vi "Mystery VI.vi"(4 "Old X-Axis":i32, 6 "Old Pin":bool[](array[boolean]), 7 "X-Axis":i32, 9 "Pin":bool[](array[boolean]), 10 "Old Trace":bool[](array[boolean]), 11 "Trace":bool[](array[boolean])) -> (1 "Updated X-Axis":i32, 2 "Updated Old Pin?":bool[](array[boolean]), 3 "NeedUpdate?":bool, 5 "Updated Old Trace?":bool[](array[boolean]))   [LabVIEW 2019]
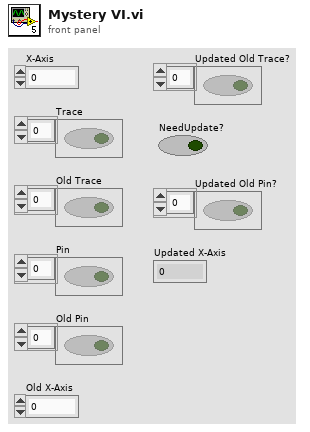
[diagram p1: front panel]
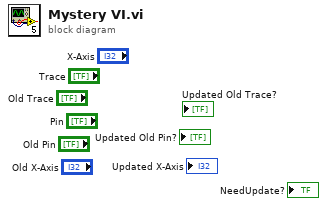
[diagram p0: block diagram]
diagram:
